vi "剖面数据_exo2.vi"(1 "data":T2={"时间"=timestamp(0 s since 1904-01-01), "测量模式"="水样测试", "数据类型"="N", "数据标识"="N", "湖面水深"=0.0, "缆绳下放长度"=0.0, "层数"=0, "Temp"=0.0, "SpCond"=0.0, "Cond"=0.0, "Sal"=0.0, "TDS"=0.0, "pH"=0.0, "pHmV"=0.0, "ORP"=0.0, "DO"=0.0, "DO%"=0.0, "Turb"=0.0, "Chla"=0.0, "Depth"=0.0}, 2 "Password":string, 3 "错误输入（无错误）":errorcluster, 4 "数据库类型":T1) -> (10 "错误输出":errorcluster)   [LabVIEW 2016]
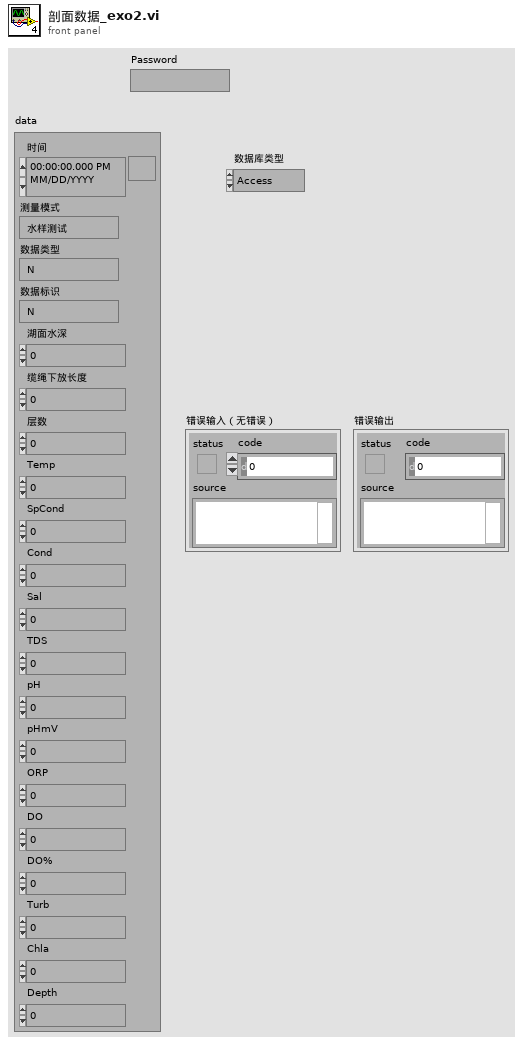
[diagram p1: front panel]
types:
  T1 = typedef "数据库类型.ctl" = enum16{"Access", "SQLite"}
  T2 = typedef "剖面数据_EXO2.ctl" = cluster{"时间":timestamp, "测量模式":string, "数据类型":string, "数据标识":string, "湖面水深":sgl, "缆绳下放长度":sgl, "层数":u16, "Temp":sgl, "SpCond":sgl, "Cond":sgl, "Sal":sgl, "TDS":sgl, "pH":sgl, "pHmV":sgl, "ORP":sgl, "DO":sgl, "DO%":sgl, "Turb":sgl, "Chla":sgl, "Depth":sgl}
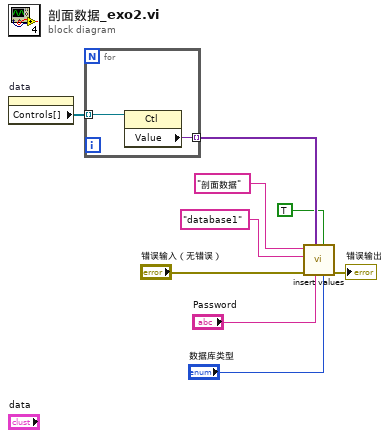
[diagram p0: block diagram]
diagram:
  n1 = property on="data" class="Clust (严格)"() -> ("Controls[]"=w9:refnum<vi>[])  [unwired: 2 in, 2 out]
  n2 = for {
    tunnel: w9 -> [w11] mode=indexing
    tunnel: [w10] -> w8 mode=indexing
    n3 = property class="Ctl"(reference=w11) -> ("Value"=w10:variant)  [unwired: 1 in, 2 out]
  }
  n4 = call "insert values.vi"("数据库类型"="数据库类型", "是否创建唯一键"=TRUE, "Password"="Password", "data"=w8, "错误输入（无错误）"="错误输入（无错误）", "database"="database1", "Tabe Name"="剖面数据") -> ("错误输出"=→"错误输出":errorcluster)  [unwired: 4 in]
